vi "PingIP.vi"(8 "error in (no error)":errorcluster, 10 "IP Address":string) -> (0 "error out":errorcluster, 1 "Ping Response":string, 2 "Response?":bool)   [LabVIEW 2020, in "Controller.lvlib"]
uses:
  Controller.lvlib
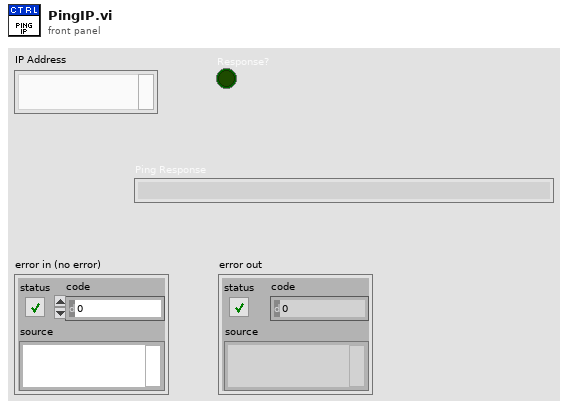
[diagram p1: front panel]
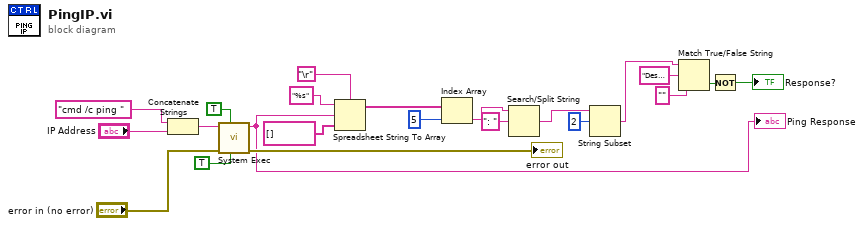
[diagram p0: block diagram]
diagram:
  n1 = Concatenate Strings("cmd /c ping " ("command line"), "IP Address") -> (w22:string)
  n2 = call <vilib>:"System Exec.vi"("run minimized? (F)"=TRUE, "wait until completion? (T)"=TRUE, "error in (no error)"="error in (no error)", "command line"=w22) -> ("error out"=→"error out":errorcluster, "standard output"=w1:string)  [unwired: 4 in, 2 out]
  "Ping Response" <- w1
  n3 = Spreadsheet String To Array(delimiter (Tab)="\r", format string="%s", spreadsheet string=w1, array type (2D Dbl)=string[] []) -> (array=w12:string[])
  n4 = Index Array(array=w12, index=5) -> (element=w7:string)
  n5 = Search/Split String(string=w7, search string/char (-)=": ") -> (match + rest of string=w10:string)  [unwired: 1 in, 2 out]
  n6 = String Subset(string=w10, offset (0)=2) -> (substring=w3:string)  [unwired: 1 in]
  n7 = Match True/False String(2:"" ("false string"), 3:"Destination host unreachable." ("true string"), 4:w3) -> (0:w5:bool)  [unwired: 1 out]
  n8 = Not(x=w5) -> (.not. x?=→"Response?":bool)
